vi "LiftGetLevel.vi"(2 "CurrentHeight":dbl) -> ()   [LabVIEW 2014, in "LiftLib.lvlib"]
uses:
  LiftLib.lvlib
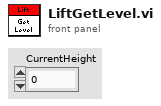
[diagram p1: front panel]
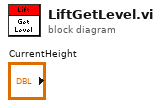
[diagram p0: block diagram]
diagram:
